vi "Monitor ConstantSet (PTC).vi"(8 "error in (no error)":errorcluster, 10 "Address (0)":i32, 11 "VISA resource name":refnum<visa-resource-name>) -> (0 "error out":errorcluster, 2 "PTC":T1, 3 "VISA resource name out":refnum<visa-resource-name>)   [LabVIEW 2016, in "Environment Chamber.lvlib" / "Climatic Chamber.lvlib"]
doc: "<b>Constant monitor\n(P-200, P-300 controllers only)</B>\n\nReturns the specimen temperature control set point in constant setup (No.1)."
uses:
  Climatic Chamber.lvlib
  Private/Type Defs/PTC ConstSetting Cluster.ctl
  Private/Type Defs/Constant OptionParameter Enum.ctl
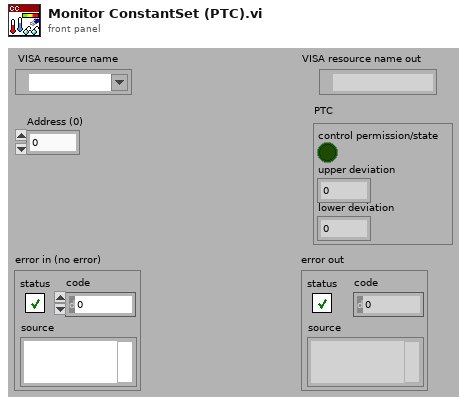
[diagram p1: front panel]
types:
  T1 = typedef "Environment Chamber.lvlib/Climatic Chamber.lvlib/PTC ConstSetting Cluster.ctl" = cluster{"control permission/state":bool, "upper deviation":dbl, "lower deviation":dbl}
  T2 = typedef "Environment Chamber.lvlib/Climatic Chamber.lvlib/Constant OptionParameter Enum.ctl" = enum16{"TEMP", "HUMI", "REF", "RELAY", "PTC"}
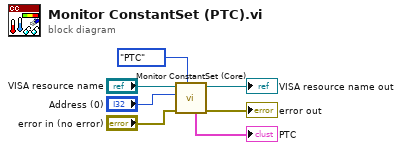
[diagram p0: block diagram]
diagram:
  n1 = call "Monitor ConstantSet (Core).vi"("Setpoint (TEMP)"=Constant_OptionParameter_Enum."PTC", "error in (no error)"="error in (no error)", "Address (0)"="Address (0)", "VISA resource name"="VISA resource name") -> ("error out"=→"error out":errorcluster, "VISA resource name out"=→"VISA resource name out":refnum<visa-resource-name>, "PTC"=→"PTC":T1)  [unwired: 2 in, 3 out]
